vi "guid.vi"() -> (0 "GUID String":string)   [LabVIEW 2019]
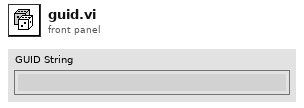
[diagram p1: front panel]
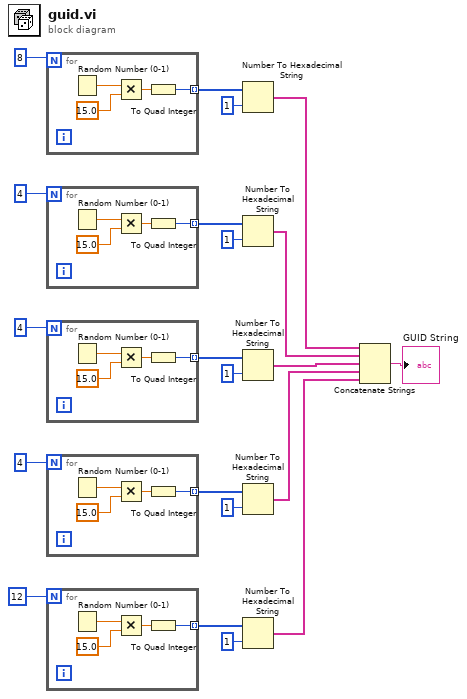
[diagram p0: block diagram]
diagram:
  n1 = for {
    N: 8 -> [_]
    tunnel: [w22] -> w20 mode=indexing
    n2 = Random Number (0-1)() -> (number: 0 to 1=w25:dbl)
    n3 = Multiply(x=w25, y=15.0) -> (x*y=w23:dbl)
    n4 = To Quad Integer(1:w23) -> (0:w22:i64)
  }
  n5 = for {
    N: 4 -> [_]
    tunnel: [w26] -> w17 mode=indexing
    n6 = Random Number (0-1)() -> (number: 0 to 1=w29:dbl)
    n7 = Multiply(x=w29, y=15.0) -> (x*y=w27:dbl)
    n8 = To Quad Integer(1:w27) -> (0:w26:i64)
  }
  n9 = for {
    N: 4 -> [_]
    tunnel: [w30] -> w14 mode=indexing
    n10 = Random Number (0-1)() -> (number: 0 to 1=w33:dbl)
    n11 = Multiply(x=w33, y=15.0) -> (x*y=w31:dbl)
    n12 = To Quad Integer(1:w31) -> (0:w30:i64)
  }
  n13 = for {
    N: 4 -> [_]
    tunnel: [w34] -> w11 mode=indexing
    n14 = Random Number (0-1)() -> (number: 0 to 1=w37:dbl)
    n15 = Multiply(x=w37, y=15.0) -> (x*y=w35:dbl)
    n16 = To Quad Integer(1:w35) -> (0:w34:i64)
  }
  n17 = for {
    N: 12 -> [_]
    tunnel: [w38] -> w8 mode=indexing
    n18 = Random Number (0-1)() -> (number: 0 to 1=w41:dbl)
    n19 = Multiply(x=w41, y=15.0) -> (x*y=w39:dbl)
    n20 = To Quad Integer(1:w39) -> (0:w38:i64)
  }
  n21 = Number To Hexadecimal String(1:i16 1 ("width (-)"), 2:w20) -> (0:w6:string[])
  n22 = Number To Hexadecimal String(1:i16 1 ("width (-)"), 2:w17) -> (0:w5:string[])
  n23 = Number To Hexadecimal String(1:i16 1 ("width (-)"), 2:w14) -> (0:w4:string[])
  n24 = Number To Hexadecimal String(1:i16 1 ("width (-)"), 2:w11) -> (0:w3:string[])
  n25 = Number To Hexadecimal String(1:i16 1 ("width (-)"), 2:w8) -> (0:w2:string[])
  n26 = Concatenate Strings(w6, w5, w4, w3, w2) -> (→"GUID String":string)
